vi "Determine Warnings.vi"() -> ()   [LabVIEW 2019]
panel:
  in  "Weather Data In":T1
  out "Error Out":errorcluster
  in  "Error In":errorcluster
  out "Weather Data Out":T1
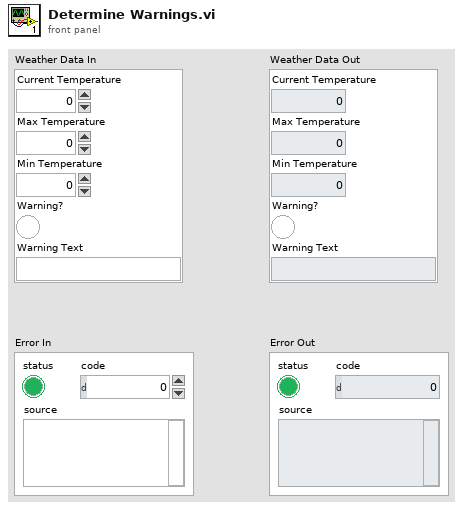
[diagram p1: front panel]
types:
  T1 = cluster{"Current Temperature":dbl, "Max Temperature":dbl, "Min Temperature":dbl, "Warning?":bool, "Warning Text":string}
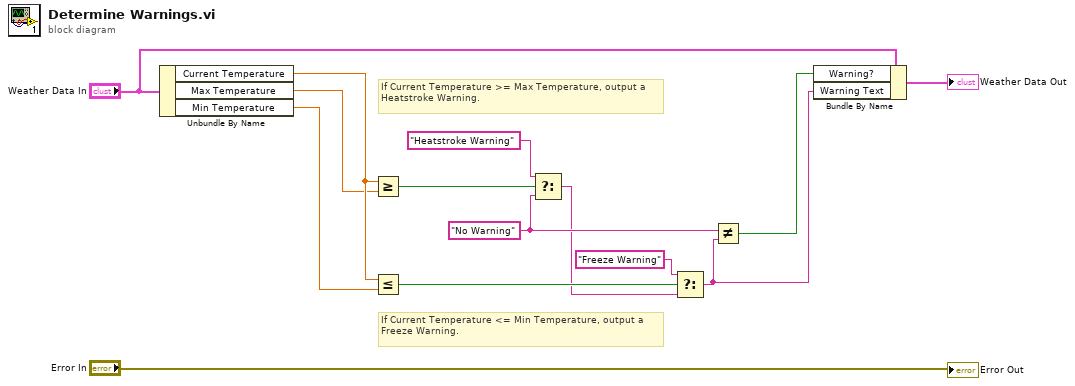
[diagram p0: block diagram]
diagram:
  w8 = "No Warning"
  # "If Current Temperature <= Min Temperature, output a Freeze Warning."
  # "If Current Temperature >= Max Temperature, output a Heatstroke Warning."
  n1 = Unbundle By Name("Weather Data In") -> ("Current Temperature"=w14:dbl, "Max Temperature"=w13:dbl, "Min Temperature"=w12:dbl)
  n2 = Greater Or Equal?(x=w14, y=w13) -> (x >= y?=w11:bool)
  n3 = Less Or Equal?(x=w14, y=w12) -> (x <= y?=w9:bool)
  n4 = Select(t="Heatstroke Warning", s=w11, f=w8) -> (s? t:f=w7:string)
  n5 = Select(t="Freeze Warning", s=w9, f=w7) -> (s? t:f=w2:string)
  n6 = Not Equal?(x=w8, y=w2) -> (x != y?=w3:bool)
  n7 = Bundle By Name(cluster="Weather Data In", "Warning?"=w3, "Warning Text"=w2) -> (→"Weather Data Out":T1)
  "Error Out" <- "Error In"
